vi "system configuration UI.vi"() -> (0 "file updated":bool)   [LabVIEW 2018]
uses:
  type defs/channelLimitControl.ctl
  type defs/limitActions.ctl
  userConfigStates.ctl
  systemConfigUIControls.ctl
  Chris VIs/data channels/parent class/Data Channel.lvclass
panel:
  in  "cancel":bool
  in  "save":bool
  in  "Tab Control":T1(tab)
  in  "pulsatorIP":string caption="Pulsator IP:"
  in  "channelConfigPath":path caption="channel configuration file"
  in  "configPath":path caption="system configuration file"
  in  "customVIPath":path caption="custom VI location"
  in  "startFolder":path caption="default data logging folder"
  in  "%":dbl
  in  "ventHowden":bool caption="Vent Howden Air"
  in  "speedFeedback":u16(ring) caption="speed feedback" items=["time", "gearbox", "Recirculation temp", "volute exit surface", "oil tank", "Inlet average", "Outlet average", "V-cone", "inlet pressure", "outlet pressure", "Motor speed", "V-cone DP", "Motor power", "Accelerometer", "Hotwire", "oil pressure", "butterfly valve position", "ball valve position", "Legacy speed", "new Vcone", "V-Cone: CR001", "pressure ratio", "Ambient pressure", "Ambient temperature"]
  in  "ballValue":u16(ring) caption="ball valve feedback" items=["time", "gearbox", "Recirculation temp", "volute exit surface", "oil tank", "Inlet average", "Outlet average", "V-cone", "inlet pressure", "outlet pressure", "Motor speed", "V-cone DP", "Motor power", "Accelerometer", "Hotwire", "oil pressure", "butterfly valve position", "ball valve position", "Legacy speed", "new Vcone", "V-Cone: CR001", "pressure ratio", "Ambient pressure", "Ambient temperature"]
  in  "butterflyValue":u16(ring) caption="butterfly valve feedback" items=["time", "gearbox", "Recirculation temp", "volute exit surface", "oil tank", "Inlet average", "Outlet average", "V-cone", "inlet pressure", "outlet pressure", "Motor speed", "V-cone DP", "Motor power", "Accelerometer", "Hotwire", "oil pressure", "butterfly valve position", "ball valve position", "Legacy speed", "new Vcone", "V-Cone: CR001", "pressure ratio", "Ambient pressure", "Ambient temperature"]
  in  "masflow":u16(ring) caption="massflow" items=["time", "gearbox", "Recirculation temp", "volute exit surface", "oil tank", "Inlet average", "Outlet average", "V-cone", "inlet pressure", "outlet pressure", "Motor speed", "V-cone DP", "Motor power", "Accelerometer", "Hotwire", "oil pressure", "butterfly valve position", "ball valve position", "Legacy speed", "new Vcone", "V-Cone: CR001", "pressure ratio", "Ambient pressure", "Ambient temperature"]
  in  "pressureRatio":u16(ring) items=["time", "gearbox", "Recirculation temp", "volute exit surface", "oil tank", "Inlet average", "Outlet average", "V-cone", "inlet pressure", "outlet pressure", "Motor speed", "V-cone DP", "Motor power", "Accelerometer", "Hotwire", "oil pressure", "butterfly valve position", "ball valve position", "Legacy speed", "new Vcone", "V-Cone: CR001", "pressure ratio", "Ambient pressure", "Ambient temperature"]
  in  "ballControl":u16(ring) caption="Ball valve control" items=["ball valve drive", "Motor Speed", "", "butterfly valve drive"]
  in  "butterflyControl":u16(ring) caption="Butterfly valve control" items=["ball valve drive", "Motor Speed", "", "butterfly valve drive"]
  in  "speedControl":u16(ring) caption="Speed control" items=["ball valve drive", "Motor Speed", "", "butterfly valve drive"]
  in  "maxSpeed":u32 caption="Hard Speed Limit (RPM):"
  in  "removeLimit":bool
  in  "addLimit":bool
  in  "channelLimits":T2[](array[typedef]) caption="Channel Limits" {"channelID" items=["time", "gearbox", "Recirculation temp", "volute exit surface", "oil tank", "Inlet average", "Outlet average", "V-cone", "inlet pressure", "outlet pressure", "Motor speed", "V-cone DP", "Motor power", "Accelerometer", "Hotwire", "oil pressure", "butterfly valve position", "ball valve position", "Legacy speed", "new Vcone", "V-Cone: CR001", "pressure ratio", "Ambient pressure", "Ambient temperature"]}
  in  "water":u16(ring) caption="Water flow:" items=["time", "gearbox", "Recirculation temp", "volute exit surface", "oil tank", "Inlet average", "Outlet average", "V-cone", "inlet pressure", "outlet pressure", "Motor speed", "V-cone DP", "Motor power", "Accelerometer", "Hotwire", "oil pressure", "butterfly valve position", "ball valve position", "Legacy speed", "new Vcone", "V-Cone: CR001", "pressure ratio", "Ambient pressure", "Ambient temperature"]
  in  "airP":u16(ring) caption="Air pressure:" items=["time", "gearbox", "Recirculation temp", "volute exit surface", "oil tank", "Inlet average", "Outlet average", "V-cone", "inlet pressure", "outlet pressure", "Motor speed", "V-cone DP", "Motor power", "Accelerometer", "Hotwire", "oil pressure", "butterfly valve position", "ball valve position", "Legacy speed", "new Vcone", "V-Cone: CR001", "pressure ratio", "Ambient pressure", "Ambient temperature"]
  in  "oilP":u16(ring) caption="Oil pressure:" items=["time", "gearbox", "Recirculation temp", "volute exit surface", "oil tank", "Inlet average", "Outlet average", "V-cone", "inlet pressure", "outlet pressure", "Motor speed", "V-cone DP", "Motor power", "Accelerometer", "Hotwire", "oil pressure", "butterfly valve position", "ball valve position", "Legacy speed", "new Vcone", "V-Cone: CR001", "pressure ratio", "Ambient pressure", "Ambient temperature"]
  in  "dataBufferLength":u16 caption="data write buffer length"
  in  "dataWriterName":string caption="cRio data NS writer name"
  in  "dataReaderName":string caption="cRio data NS reader name"
  in  "dataBufferSize":u16 caption="data Stream buffer size"
  in  "commandBufferSize":u16 caption="command buffer size"
  in  "commandReaderName":string caption="cRio command NS reader name"
  in  "commandWriterName":string caption="cRio command NS writer name"
  in  "errorBufferSize":u16 caption="error stream buffer size"
  in  "errorWriterName":string caption="cRIO error NS writer name"
  in  "errorReaderName":string caption="cRIO error NS reader name"
  in  "scanPeriod":u16 caption="scanivalve scan period (ms)"
  in  "scanivalveIP":string caption="scanivalve IP address"
  in  "incidentLogfile":path caption="error logfile path"
  in  "RTIP":string caption="cRio IP address"
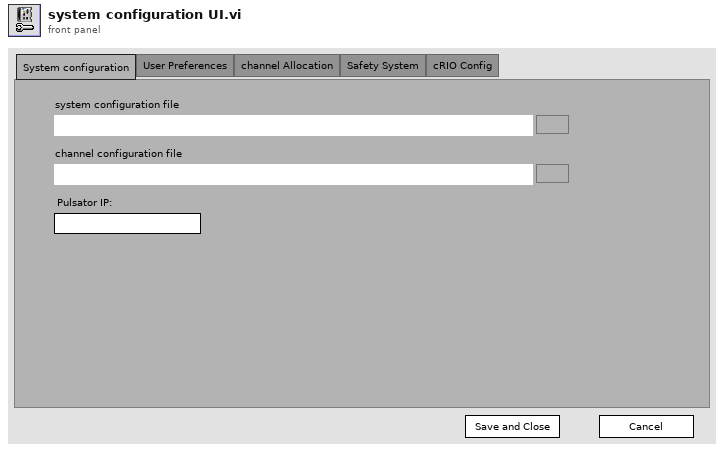
[diagram p1: front panel]
types:
  T1 = enum32{"System configuration", "User Preferences", "channel Allocation", "Safety System", "cRIO Config"}
  T2 = typedef "channelLimitControl.ctl" = cluster{"channelID":u16, "Enabled":bool, "warnValue":dbl, "limitValue":dbl, "Invert":bool, "limitAction":T3}
  T3 = typedef "limitActions.ctl" = enum16{"stop", "shutdown", "ignore"}
  T4 = typedef "systemConfigUIControls.ctl" = cluster{"allControls":cluster{"feedbackChannels":cluster{"butterfly":refnum<vi>, "ball":refnum<vi>, "massflow":refnum<vi>, "pressureRatio":refnum<vi>, "airP":refnum<vi>, "water":refnum<vi>, "oilP":refnum<vi>, "speed":refnum<vi>}, "controlChannels":cluster{"butterflyControl":refnum<vi>, "ballControl":refnum<vi>, "speedControl":refnum<vi>}, "channelLimits":refnum<vi>, "pulsatorIP":string}, "allValues":cluster{"feedback":cluster{"butterfly":u16, "ball":u16, "massflow":u16, "pressureRatio":u16, "airP":u16, "water":u16, "oilP":u16, "speed":u16}, "paths":cluster{"channelConfig":path, "systemConfig":path, "incidentLogfile":path, "startFolder":path, "customVI":path}, "RT":cluster{"RTIP":string, "errorReaderName":string, "errorWriterName":string, "errorBufferSize":u16, "commandWriterName":string, "commandReaderName":string, "commandBufferSize":u16, "dataBufferSize":u16, "dataReaderName":string, "dataWriterName":string, "dataBufferLength":u16, "scanivalveIP":string, "scanPeriod":u16}, "controls":cluster{"butterflyControl":u16, "ballControl":u16, "speedControl":u16}, "safetyLimits":cluster{"channelLimits":T2[], "maxSpeed":u32}, "Howden":cluster{"howdenAir":bool, "howden%":dbl}}, "variables":cluster{"feedbackChannelIDs":u16[], "controlChannelIDs":u16[], "channelsArray":refnum<class "Data Channel.lvclass">[]}}
  T5 = typedef "userConfigStates.ctl" = enum16{"wait", "init", "updateControls", "save", "cancel"}
  T6 = cluster{"speedFeedback":u16, "ballValue":u16, "butterflyValue":u16, "masflow":u16, "pressureRatio":u16, "ballControl":u16, "butterflyControl":u16, "speedControl":u16, "oilP":u16}
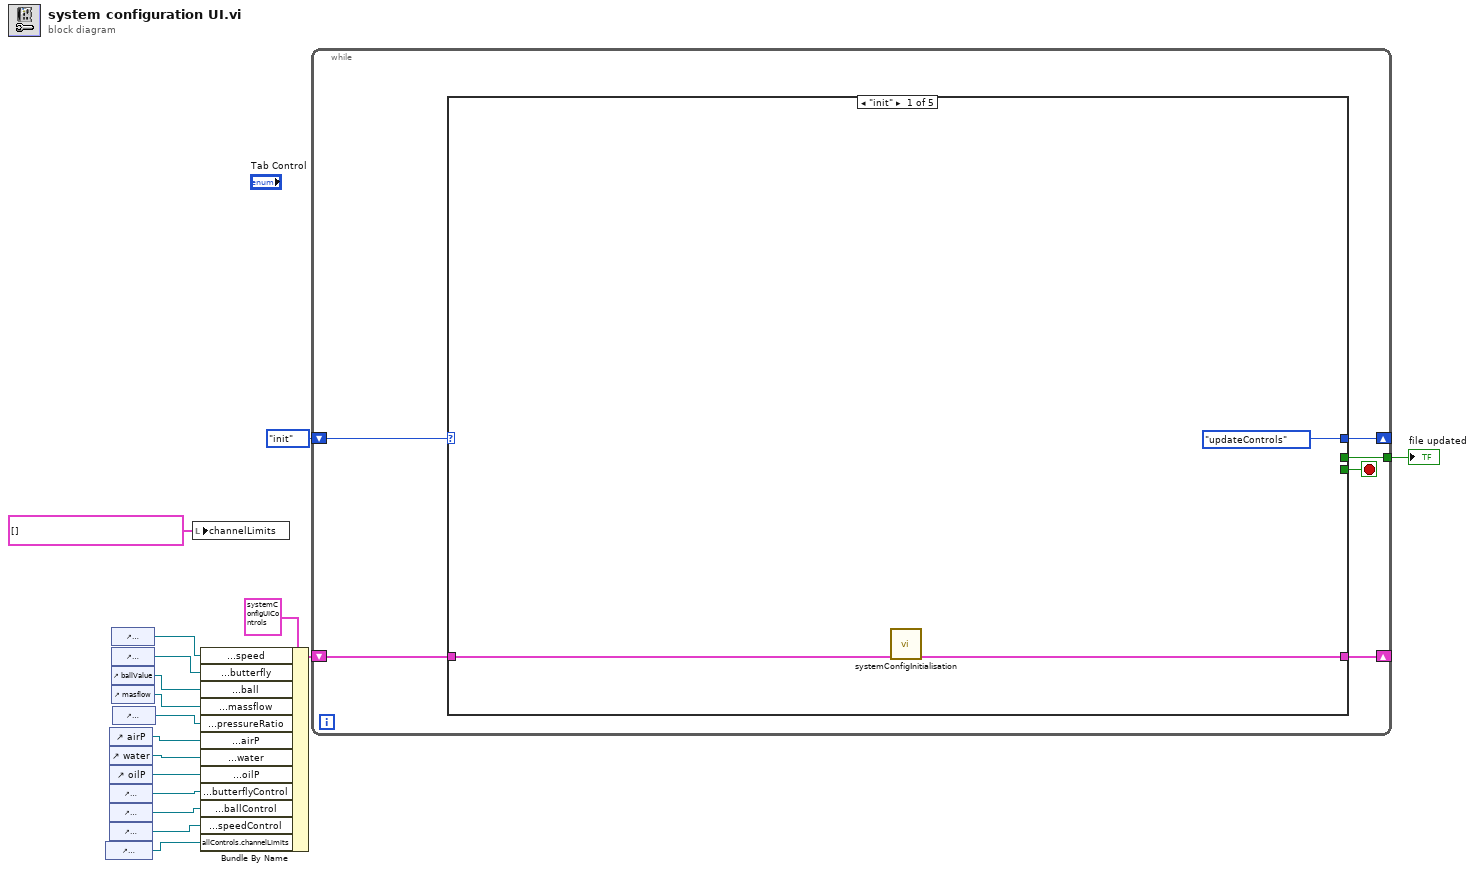
[diagram p0: block diagram]
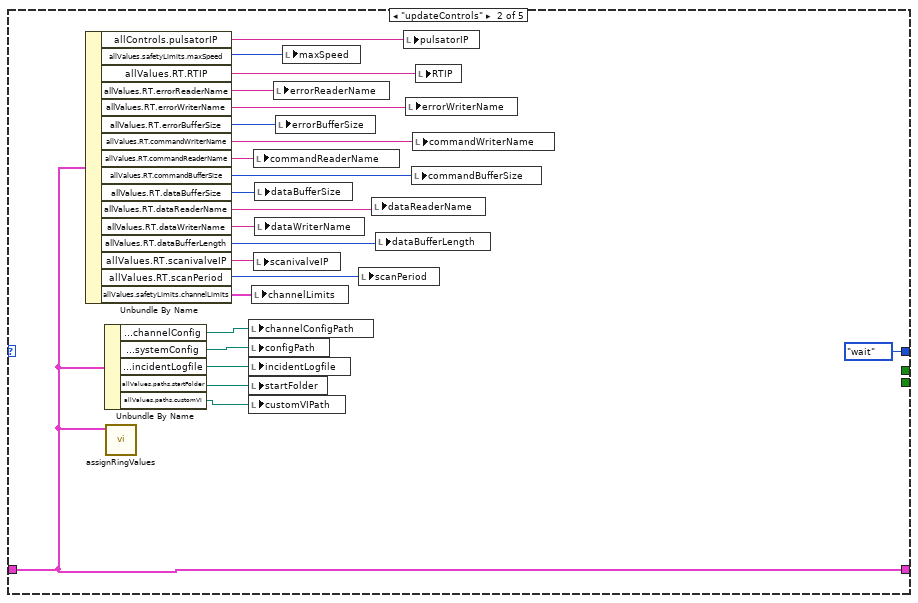
[diagram p2: hidden frame]
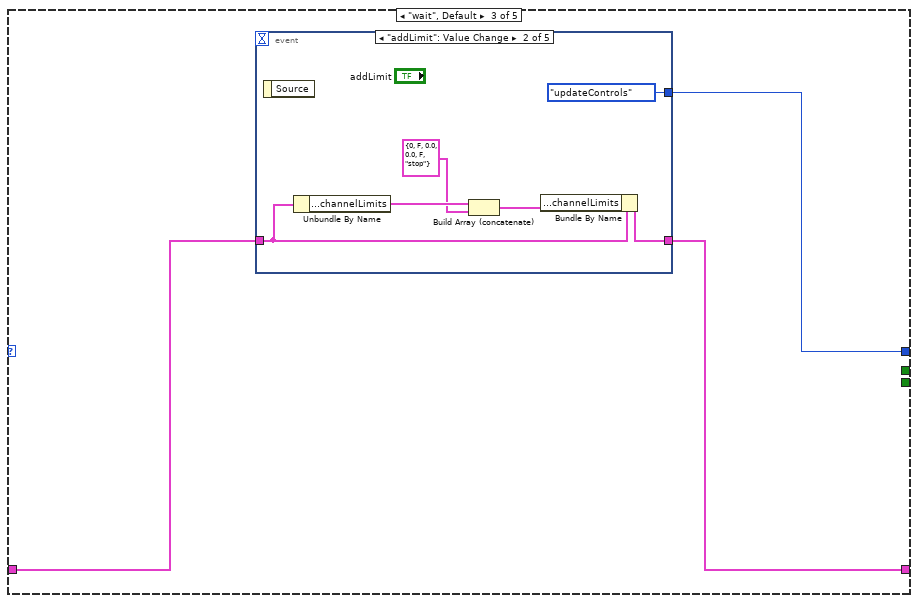
[diagram p3: hidden frame]
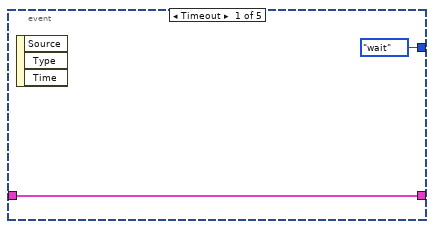
[diagram p4: hidden frame]
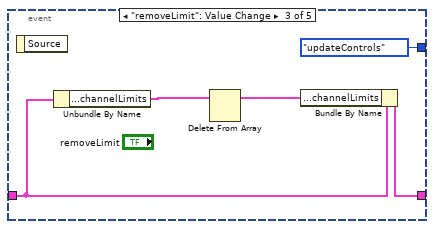
[diagram p5: hidden frame]
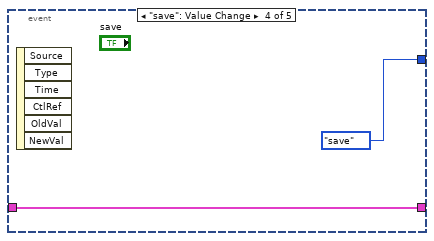
[diagram p6: hidden frame]
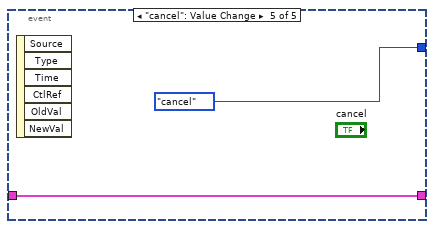
[diagram p7: hidden frame]
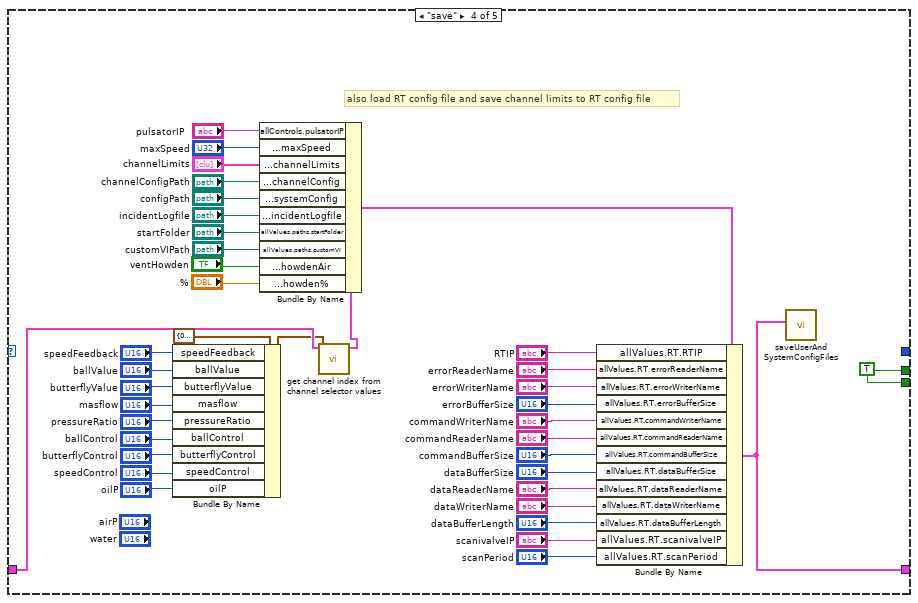
[diagram p8: hidden frame]
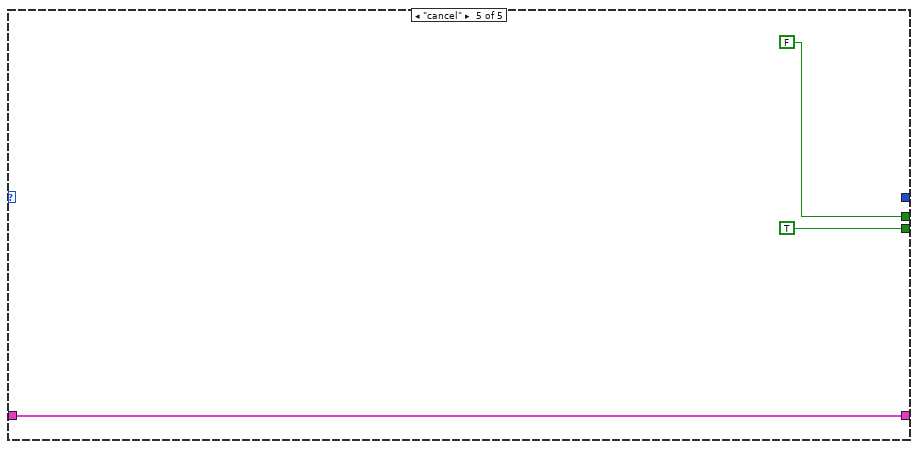
[diagram p9: hidden frame]
diagram:
  n1 = control-ref of="channelLimits"() -> (w3:refnum<vi>)
  n2 = control-ref of="airP"() -> (w10:refnum<vi>)
  n3 = control-ref of="water"() -> (w9:refnum<vi>)
  n4 = control-ref of="oilP"() -> (w8:refnum<vi>)
  n5 = control-ref of="butterflyControl"() -> (w7:refnum<vi>)
  n6 = control-ref of="ballControl"() -> (w6:refnum<vi>)
  n7 = control-ref of="speedControl"() -> (w5:refnum<vi>)
  n8 = control-ref of="speedFeedback"() -> (w4:refnum<vi>)
  n9 = control-ref of="butterflyValue"() -> (w13:refnum<vi>)
  n10 = control-ref of="ballValue"() -> (w12:refnum<vi>)
  n11 = control-ref of="masflow"() -> (w11:refnum<vi>)
  n12 = control-ref of="pressureRatio"() -> (w1:refnum<vi>)
  n13 = local write "channelLimits"(T2[] [] ("channelLimits")) -> ()
  n14 = Bundle By Name(cluster=T4 {"allControls"={"feedbackChannels"={"butterfly"=refnum, "ball"=refnum, "massflow"=refnum, "pressureRatio"=refnum, "airP"=refnum, "water"=refnum, "oilP"=refnum, "speed"=refnum}, "controlChannels"={"butterflyControl"=refnum, "ballControl"=refnum, "speedControl"=refnum}, "channelLimits"=refnum, "pulsatorIP"=""}, "allValues"={"feedback"={"butterfly"=0, "ball"=0, "massflow"=0, "pressureRatio"=0, "airP"=0, "water"=0, "oilP"=0, "speed"=0}, "paths"={"channelConfig"=path "", "systemConfig"=path "", "incidentLogfile"=path "", "startFolder"=path "", "customVI"=path ""}, "RT"={"RTIP"="", "errorReaderName"="", "errorWriterName"="", "errorBufferSize"=0, "commandWriterName"="", "commandReaderName"="", "commandBufferSize"=0, "dataBufferSize"=0, "dataReaderName"="", "dataWriterName"="", "dataBufferLength"=0, "scanivalveIP"="", "scanPeriod"=0}, "controls"={"butterflyControl"=0, "ballControl"=0, "speedControl"=0}, "safetyLimits"={"channelLimits"=[], "maxSpeed"=0}, "Howden"={"howdenAir"=FALSE, "howden%"=0.0}}, "variables"={"feedbackChannelIDs"=[], "controlChannelIDs"=[], "channelsArray"=[]}} ("controls"), "allControls.feedbackChannels.speed"=w4, "allControls.feedbackChannels.butterfly"=w13, "allControls.feedbackChannels.ball"=w12, "allControls.feedbackChannels.massflow"=w11, "allControls.feedbackChannels.pressureRatio"=w1, "allControls.feedbackChannels.airP"=w10, "allControls.feedbackChannels.water"=w9, "allControls.feedbackChannels.oilP"=w8, "allControls.controlChannels.butterflyControl"=w7, "allControls.controlChannels.ballControl"=w6, "allControls.controlChannels.speedControl"=w5, "allControls.channelLimits"=w3) -> (w14:T4)
  n15 = while {
    shift-right: [w22] -> _
    shift-left: userConfigStates."init" -> [w23]
    tunnel: [w21] -> w16
    shift-right: [w18] -> _
    shift-left: w14 -> [w19]
    stop <- w20 stop-if-true
    n16 = case shown="\"init\"" w23 {
      tunnel: [userConfigStates."updateControls" userConfigStates."wait" w52 _ _] -> w22
      tunnel: [_ _ _ w108 FALSE] -> w21
      tunnel: [_ _ _ w108 TRUE] -> w20
      tunnel: w19 -> [w26 w45 w51 w85 w109]
      tunnel: [w25 w45 w50 w107 w109] -> w18
      frame "init" {
        n17 = call "systemConfigInitialisation.vi"("configData"=w26) -> ("configData out"=w25:T4)  [unwired: 10 in]
      }
      frame "updateControls" {
        n18 = Unbundle By Name(w45) -> ("allControls.pulsatorIP"=w27:string, "allValues.safetyLimits.maxSpeed"=w28:u32, "allValues.RT.RTIP"=w35:string, "allValues.RT.errorReaderName"=w34:string, "allValues.RT.errorWriterName"=w44:string, "allValues.RT.errorBufferSize"=w43:u16, "allValues.RT.commandWriterName"=w42:string, "allValues.RT.commandReaderName"=w41:string, "allValues.RT.commandBufferSize"=w40:u16, "allValues.RT.dataBufferSize"=w39:u16, "allValues.RT.dataReaderName"=w38:string, "allValues.RT.dataWriterName"=w37:string, "allValues.RT.dataBufferLength"=w36:u16, "allValues.RT.scanivalveIP"=w33:string, "allValues.RT.scanPeriod"=w32:u16, "allValues.safetyLimits.channelLimits"=w30:T2[])
        n19 = Unbundle By Name(w45) -> ("allValues.paths.channelConfig"=w46:path, "allValues.paths.systemConfig"=w47:path, "allValues.paths.incidentLogfile"=w49:path, "allValues.paths.startFolder"=w48:path, "allValues.paths.customVI"=w29:path)
        n20 = call "assignRingValues.vi"("controls"=w45) -> ()  [unwired: 11 in]
        n21 = local write "channelConfigPath"(w46) -> ()
        n22 = local write "configPath"(w47) -> ()
        n23 = local write "incidentLogfile"(w49) -> ()
        n24 = local write "startFolder"(w48) -> ()
        n25 = local write "customVIPath"(w29) -> ()
        n26 = local write "channelLimits"(w30) -> ()
        n27 = local write "commandReaderName"(w41) -> ()
        n28 = local write "scanivalveIP"(w33) -> ()
        n29 = local write "dataBufferSize"(w39) -> ()
        n30 = local write "dataWriterName"(w37) -> ()
        n31 = local write "errorReaderName"(w34) -> ()
        n32 = local write "errorBufferSize"(w43) -> ()
        n33 = local write "maxSpeed"(w28) -> ()
        n34 = local write "scanPeriod"(w32) -> ()
        n35 = local write "dataReaderName"(w38) -> ()
        n36 = local write "dataBufferLength"(w36) -> ()
        n37 = local write "pulsatorIP"(w27) -> ()
        n38 = local write "errorWriterName"(w44) -> ()
        n39 = local write "commandBufferSize"(w40) -> ()
        n40 = local write "commandWriterName"(w42) -> ()
        n41 = local write "RTIP"(w35) -> ()
      }
      frame "wait", Default {
        n42 = event shown="[1] \"addLimit\": Value Change" {
          selector: _ -> [_ _ _ _ _]
          dyn-events: _ -> [_ _ _ _ _]
          timeout: _ -> [_ _ _ _ _]
          tunnel: [userConfigStates."wait" userConfigStates."updateControls" userConfigStates."updateControls" userConfigStates."save" userConfigStates."cancel"] -> w52
          tunnel: [w54 w59 w64 w66 w68] -> w50
          tunnel: w51 -> [w54 w60 w65 w66 w68]
          event Timeout {
            n43 = event-data() -> ()  [unwired: 1 in, 3 out]
          }
          event "addLimit": Value Change {
            n44 = event-data() -> ()  [unwired: 1 in, 1 out]
            n45 = Unbundle By Name(w60) -> ("allValues.safetyLimits.channelLimits"=w58:T2[])
            n46 = Build Array (concatenate)(w58, T2 {"channelID"=0, "Enabled"=FALSE, "warnValue"=0.0, "limitValue"=0.0, "Invert"=FALSE, "limitAction"=enum."stop"} ("Temperature monitoring")) -> (w57:T2[])
            n47 = Bundle By Name(cluster=w60, "allValues.safetyLimits.channelLimits"=w57) -> (w59:T4)
          }
          event "removeLimit": Value Change {
            n48 = event-data() -> ()  [unwired: 1 in, 1 out]
            n49 = Unbundle By Name(w65) -> ("allValues.safetyLimits.channelLimits"=w63:T2[])
            n50 = Delete From Array(array=w63) -> (array with subset deleted=w62:T2[])  [unwired: 2 in, 1 out]
            n51 = Bundle By Name(cluster=w65, "allValues.safetyLimits.channelLimits"=w62) -> (w64:T4)
          }
          event "save": Value Change {
            n52 = event-data() -> ()  [unwired: 1 in, 6 out]
          }
          event "cancel": Value Change {
            n53 = event-data() -> ()  [unwired: 1 in, 6 out]
          }
        }
      }
      frame "save" {
        w108 = TRUE
        # "also load RT config file and save channel limits to RT config file"
        n54 = Bundle By Name(cluster=T6 {"speedFeedback"=0, "ballValue"=0, "butterflyValue"=0, "masflow"=0, "pressureRatio"=0, "ballControl"=0, "butterflyControl"=0, "speedControl"=0, "oilP"=0} ("channelSelection"), "speedFeedback"="speedFeedback", "ballValue"="ballValue", "butterflyValue"="butterflyValue", "masflow"="masflow", "pressureRatio"="pressureRatio", "ballControl"="ballControl", "butterflyControl"="butterflyControl", "speedControl"="speedControl", "oilP"="oilP") -> (w83:T6)
        n55 = call "get channel index from channel selector values.vi"("channelSelection"=w83, "controls in"=w85) -> ("controls out"=w93:T4)  [unwired: 9 in]
        n56 = Bundle By Name(cluster=w93, "allControls.pulsatorIP"="pulsatorIP", "allValues.safetyLimits.maxSpeed"="maxSpeed", "allValues.safetyLimits.channelLimits"="channelLimits", "allValues.paths.channelConfig"="channelConfigPath", "allValues.paths.systemConfig"="configPath", "allValues.paths.incidentLogfile"="incidentLogfile", "allValues.paths.startFolder"="startFolder", "allValues.paths.customVI"="customVIPath", "allValues.Howden.howdenAir"="ventHowden", "allValues.Howden.howden%"="%") -> (w92:T4)
        n57 = Bundle By Name(cluster=w92, "allValues.RT.RTIP"="RTIP", "allValues.RT.errorReaderName"="errorReaderName", "allValues.RT.errorWriterName"="errorWriterName", "allValues.RT.errorBufferSize"="errorBufferSize", "allValues.RT.commandWriterName"="commandWriterName", "allValues.RT.commandReaderName"="commandReaderName", "allValues.RT.commandBufferSize"="commandBufferSize", "allValues.RT.dataBufferSize"="dataBufferSize", "allValues.RT.dataReaderName"="dataReaderName", "allValues.RT.dataWriterName"="dataWriterName", "allValues.RT.dataBufferLength"="dataBufferLength", "allValues.RT.scanivalveIP"="scanivalveIP", "allValues.RT.scanPeriod"="scanPeriod") -> (w107:T4)
        n58 = call "saveUserAnd SystemConfigFiles.vi"("controls"=w107) -> ()  [unwired: 11 in]
      }
      frame "cancel" {
      }
    }
  }
  "file updated" <- w16
